vi "Main.vi"() -> ()   [LabVIEW 2020]
uses:
  subVis/globalVariable.vi
  <vilib>/addons/zeromq/zeromq.lvlib
panel:
  out "output cluster":T1
  # "(-300 tot -350) Z:"
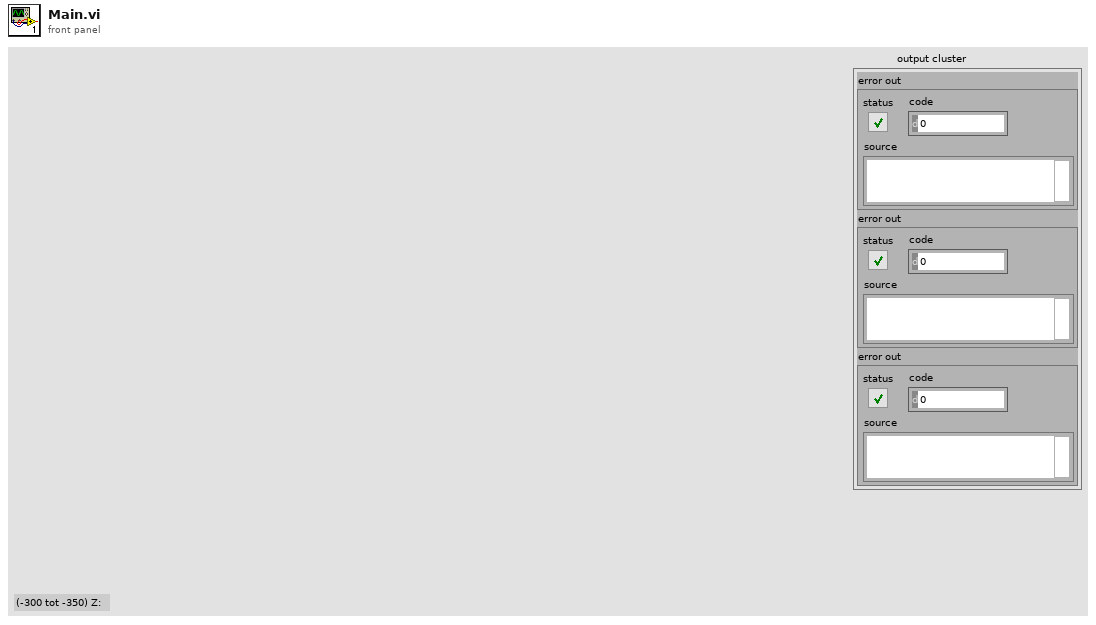
[diagram p1: front panel]
types:
  T1 = cluster{"error out":errorcluster, "error out":errorcluster, "error out":errorcluster}
  T2 = typedef "states.ctl" = enum16{"Idle", "Home", "Move", "DisableAxis", "HomePosition", "Stop"}
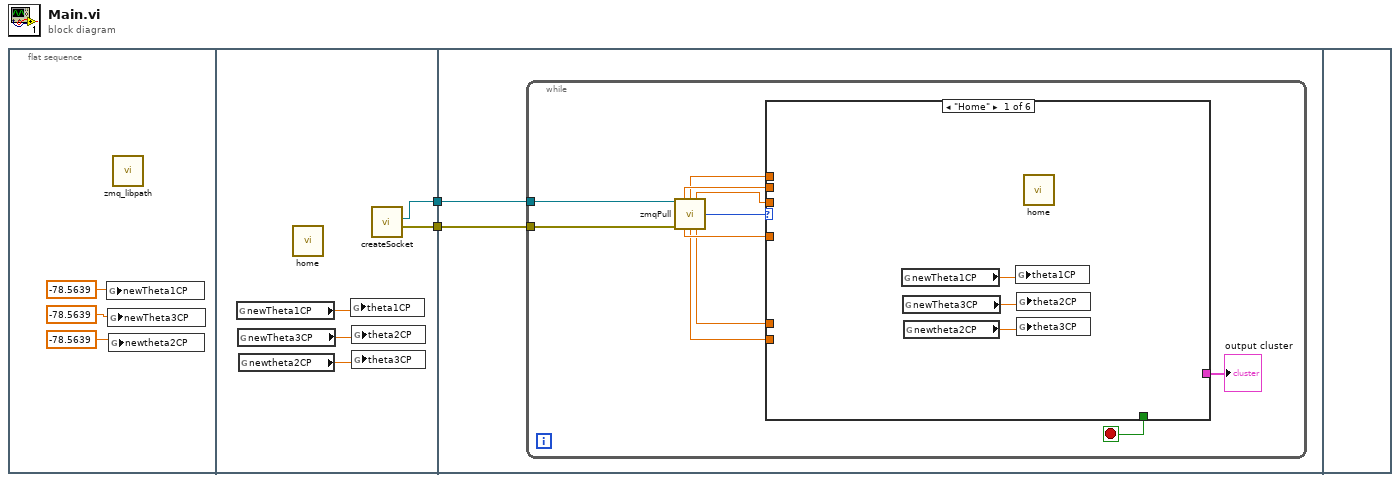
[diagram p0: block diagram]
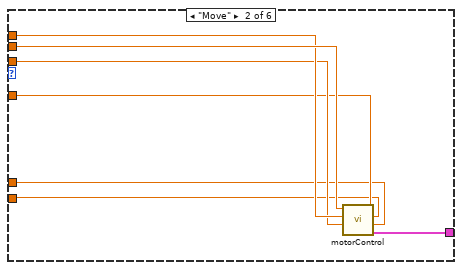
[diagram p2: hidden frame]
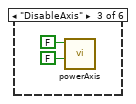
[diagram p3: hidden frame]
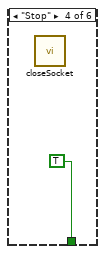
[diagram p4: hidden frame]
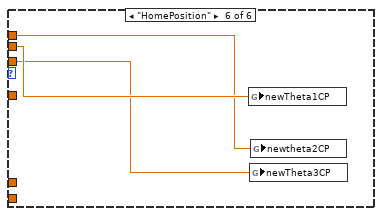
[diagram p6: hidden frame]
diagram:
  n1 = flat-sequence {
    tunnel: [w10] -> w2
    tunnel: [w9] -> w1
    tunnel: w2 -> [w12]
    tunnel: w1 -> [w11]
    frame #0 {
      n2 = global write "globalVariable.vi" "newTheta1CP"(-78.5639 ("theta1CP")) -> ()
      n3 = global write "globalVariable.vi" "newTheta3CP"(-78.5639 ("theta1CP")) -> ()
      n4 = global write "globalVariable.vi" "newtheta2CP"(-78.5639 ("theta1CP")) -> ()
      n5 = call <vilib>:"zmq_libpath.vi"() -> ()  [unwired: 1 out]
    }
    frame #1 {
      n6 = global read "globalVariable.vi" "newTheta1CP"() -> (w8:dbl)
      n7 = global read "globalVariable.vi" "newTheta3CP"() -> (w7:dbl)
      n8 = global read "globalVariable.vi" "newtheta2CP"() -> (w6:dbl)
      n9 = call "home.vi"() -> ()  [unwired: 12 in]
      n10 = global write "globalVariable.vi" "theta1CP"(w8) -> ()
      n11 = global write "globalVariable.vi" "theta2CP"(w7) -> ()
      n12 = global write "globalVariable.vi" "theta3CP"(w6) -> ()
      n13 = call "createSocket.vi"() -> ("error out"=w10:errorcluster, "socket out"=w9:refnum<class "zmq_socket.lvclass">)  [unwired: 9 in, 1 out]
    }
    frame #2 {
      n14 = while {
        tunnel: w12 -> [w20]
        tunnel: w11 -> [w21]
        stop <- w23 stop-if-true
        n15 = call "zmqPull.vi"("socket in"=w21, "error in"=w20) -> ("X"=w18:dbl, "Y"=w17:dbl, "Z"=w16:dbl, "state"=w19:T2, "velocity"=w15:dbl, "accel."=w14:dbl, "deccel."=w13:dbl)  [unwired: 5 in, 2 out]
        n16 = case shown="\"Home\"" w19 {
          tunnel: [_ _ _ TRUE _ _] -> w23
          tunnel: [_ w33 _ _ _ _] -> w22
          tunnel: w18 -> [_ w32 _ _ _ w39]
          tunnel: w17 -> [_ w31 _ _ _ w38]
          tunnel: w16 -> [_ w30 _ _ _ w37]
          tunnel: w15 -> [_ w29 _ _ _ _]
          tunnel: w14 -> [_ w28 _ _ _ _]
          tunnel: w13 -> [_ w27 _ _ _ _]
          frame "Home" {
            n17 = global read "globalVariable.vi" "newTheta1CP"() -> (w26:dbl)
            n18 = global read "globalVariable.vi" "newTheta3CP"() -> (w25:dbl)
            n19 = global read "globalVariable.vi" "newtheta2CP"() -> (w24:dbl)
            n20 = global write "globalVariable.vi" "theta1CP"(w26) -> ()
            n21 = global write "globalVariable.vi" "theta2CP"(w25) -> ()
            n22 = global write "globalVariable.vi" "theta3CP"(w24) -> ()
            n23 = call "home.vi"() -> ()  [unwired: 12 in]
          }
          frame "Move" {
            n24 = call "motorControl.vi"("deceleration"=w27, "acceleration"=w28, "velocity"=w29, "Z"=w30, "Y"=w31, "X"=w32) -> ("output cluster"=w33:T1)  [unwired: 5 in]
          }
          frame "DisableAxis" {
            n25 = call "powerAxis.vi"("enable drive"=FALSE, "enable axis"=FALSE) -> ()  [unwired: 10 in]
          }
          frame "Stop" {
            n26 = call "closeSocket.vi"() -> ()  [unwired: 12 in]
          }
          frame "Idle" {
          }
          frame "HomePosition" {
            n27 = global write "globalVariable.vi" "newTheta1CP"(w39) -> ()
            n28 = global write "globalVariable.vi" "newTheta3CP"(w37) -> ()
            n29 = global write "globalVariable.vi" "newtheta2CP"(w38) -> ()
          }
        }
        "output cluster" <- w22
      }
    }
    frame #3 {
    }
  }
